vi "LaserRW.vi"(3 "error in (no error)":errorcluster, 4 "buffer à écrire":string="V?", 5 "Nom de ressource VISA":refnum<visa-resource-name>) -> (0 "error out":errorcluster, 1 "buffer lu":string, 2 "Nom de ressource VISA en sortie":refnum<visa-resource-name>)   [LabVIEW 2011]
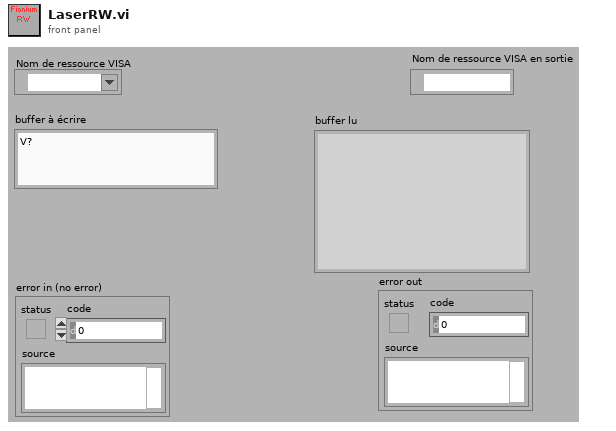
[diagram p1: front panel]
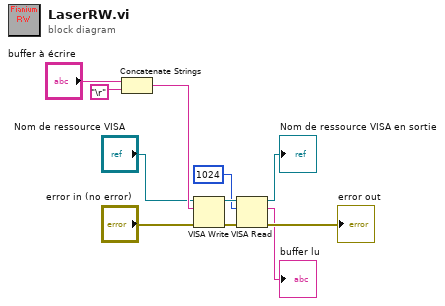
[diagram p0: block diagram]
diagram:
  n1 = Concatenate Strings("buffer à écrire", "\r") -> (w11:string)
  n2 = VISA Write(VISA resource name="Nom de ressource VISA", write buffer=w11, error in (no error)="error in (no error)") -> (VISA resource name out=w9:refnum<visa-resource-name>, error out=w8:errorcluster)  [unwired: 1 out]
  n3 = VISA Read(VISA resource name=w9, byte count=u32 1024 ("nombre d'octets"), error in (no error)=w8) -> (VISA resource name out=→"Nom de ressource VISA en sortie":refnum<visa-resource-name>, read buffer=→"buffer lu":string, error out=→"error out":errorcluster)  [unwired: 1 out]
